vi "SubtractionHandler_Create.vi"(8 "Error In":errorcluster, 11 "reference in":refnum<class "SubtractionHandler.lvclass">) -> (0 "Error Out":errorcluster, 3 "reference out":refnum<class "SubtractionHandler.lvclass">)   [LabVIEW 2020, in "SubtractionHandler.lvclass"]
uses:
  SubtractionHandler.lvclass
  C:/Projects/OpenGDS_DesignPatterns/ChainOfResponsibility1/BaseHandler_class/BaseHandler.lvclass
  BaseHandler_class/BaseHandler.lvclass
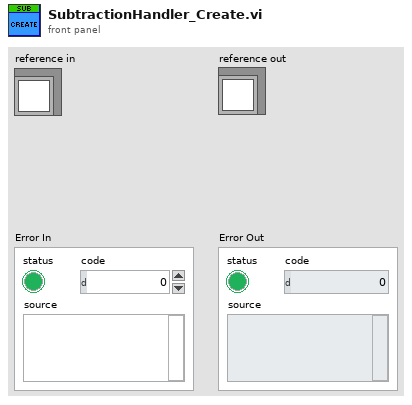
[diagram p1: front panel]
types:
  T1 = typedef "SubtractionHandler.lvclass/ObjectAttributes.ctl" = cluster{"None":bool}
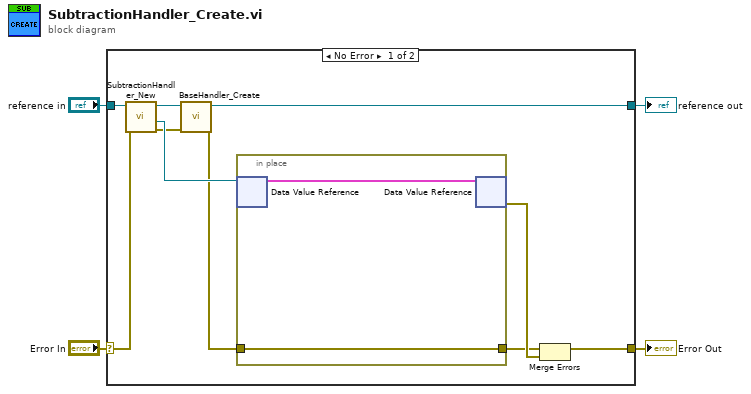
[diagram p0: block diagram]
diagram:
  n1 = case shown="No Error" "Error In" {
    selector: "Error In" -> [w10 w18]
    tunnel: [w8 w18] -> w3
    tunnel: "reference in" -> [w12 w17]
    tunnel: [w7 w17] -> w1
    frame No Error {
      n2 = call "SubtractionHandler_New.vi"("error in (no error)"=w10, "reference in"=w12) -> ("error out"=w11:errorcluster, "DVRRefOut"=w14:refnum<data-value>, "reference out"=w13:refnum<class "SubtractionHandler.lvclass">)  [unwired: 6 in, 1 out]
      n3 = call "BaseHandler_Create.vi"("Error In"=w11, "reference in"=w13) -> ("Error Out"=w6:errorcluster, "reference out"=w7:refnum<class "SubtractionHandler.lvclass">)  [unwired: 8 in]
      n4 = in-place {
        in-place-border: w6 -> [w16]
        in-place-border: [w16] -> w5
        n5 = in-place-dvr #1(w14) -> (w15:T1)  [unwired: 1 out]
        n6 = in-place-dvr #1(w15) -> (w9:errorcluster)  [unwired: 1 out]
      }
      n7 = Merge Errors(w5, w9) -> (w8:errorcluster)
    }
    frame Error {
    }
  }
  "Error Out" <- w3
  "reference out" <- w1
